vi "CursVisMidRange.vi"(11 "XYGraph in":refnum<vi>) -> ()   [LabVIEW 2014]
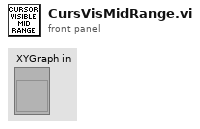
[diagram p1: front panel]
types:
  T1 = typedef "LVRangeTypeDef.ctl" = cluster{"Minimum":dbl, "Maximum":dbl, "Increment":dbl, "Minor Increment":dbl, "Start":dbl}
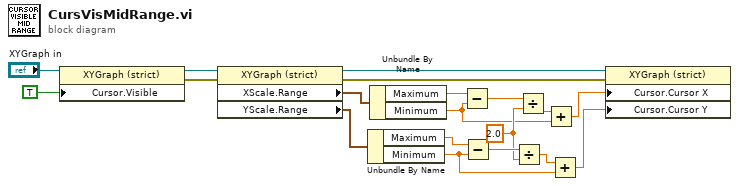
[diagram p0: block diagram]
diagram:
  w11 = 2.0 ("y")
  n1 = property on="Property Node" class="XYGraph (strict)"(reference="XYGraph in", "Cursor.Visible"=TRUE) -> (error out=w18:errorcluster)  [unwired: 1 in, 1 out]
  n2 = property on="Property Node" class="XYGraph (strict)"(reference="XYGraph in", error in=w18) -> (reference out=w2:refnum<vi>, error out=w4:errorcluster, "XScale.Range"=w16:T1, "YScale.Range"=w17:T1)
  n3 = Unbundle By Name(w17) -> ("Maximum"=w15:dbl, "Minimum"=w7:dbl)
  n4 = Unbundle By Name(w16) -> ("Maximum"=w14:dbl, "Minimum"=w9:dbl)
  n5 = Subtract(x=w14, y=w9) -> (x-y=w13:dbl)
  n6 = Subtract(x=w15, y=w7) -> (x-y=w12:dbl)
  n7 = Divide(x=w12, y=w11) -> (x/y=w8:dbl)
  n8 = Divide(x=w13, y=w11) -> (x/y=w10:dbl)
  n9 = Add(x=w10, y=w9) -> (x+y=w6:dbl)
  n10 = Add(x=w8, y=w7) -> (x+y=w5:dbl)
  n11 = property on="Property Node" class="XYGraph (strict)"(reference=w2, error in=w4, "Cursor.Cursor X"=w6, "Cursor.Cursor Y"=w5) -> ()  [unwired: 2 out]
